vi "HDrive.Hashtag.vi"(2 "Percentage":dbl, 3 "Heading":dbl, 4 "X Input":dbl, 5 "Y Input":dbl) -> (0 "X Output":dbl, 1 "Y Output":dbl)   [LabVIEW 2014]
panel:
  out "Y-State":u16(ring) items=["Negative", "Positive"]
  out "X-State":u16(ring) items=["Negative", "Positive"]
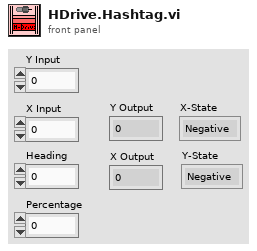
[diagram p1: front panel]
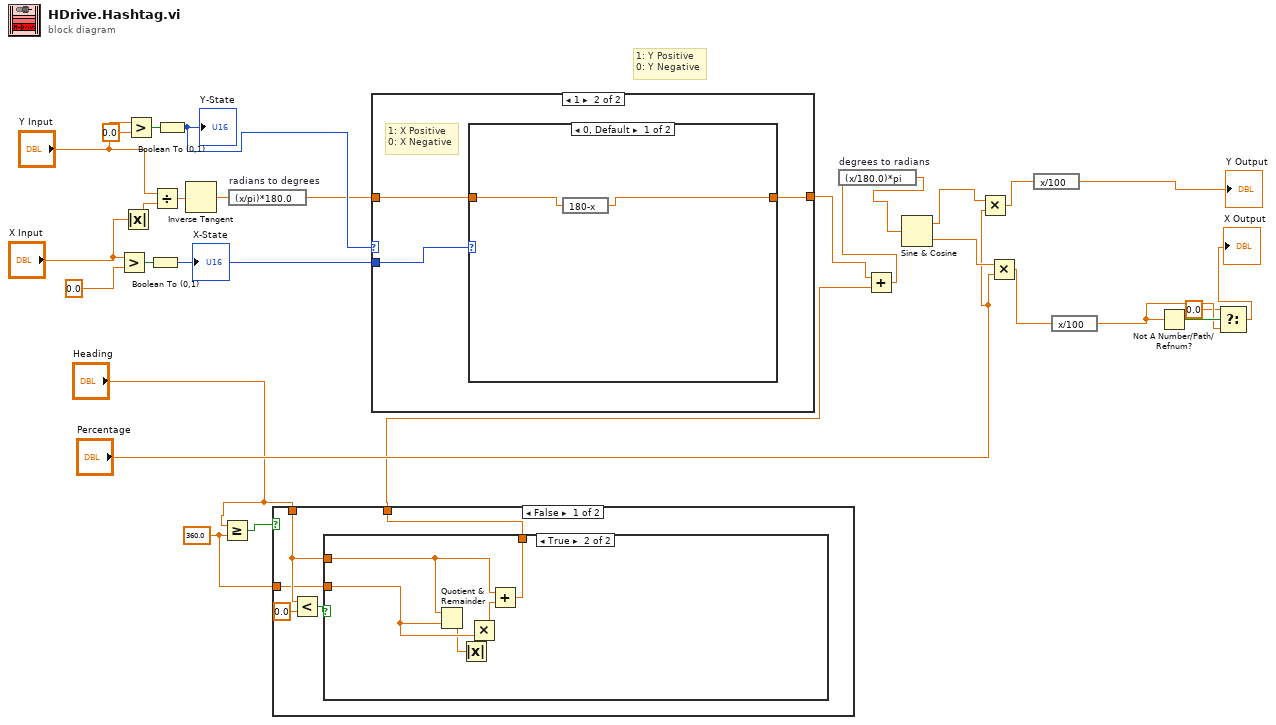
[diagram p0: block diagram]
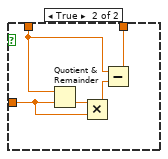
[diagram p3: hidden frame]
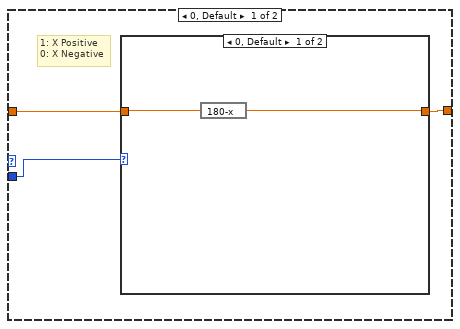
[diagram p4: hidden frame]
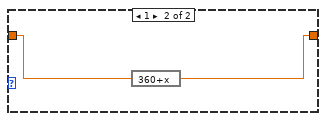
[diagram p5: hidden frame]
diagram:
  w8 = 360.0 ("y")
  # "1: Y Positive\n0: Y Negative"
  n1 = Greater?(x="X Input", y=0.0) -> (0:w27:bool)
  n2 = Absolute Value(x="X Input") -> (abs(x)=w28:dbl)
  n3 = Greater?(x="Y Input", y=0.0) -> (0:w24:bool)
  n4 = Boolean To (0,1)(Boolean=w27) -> (0, 1=w21:i16)
  "X-State" <- w21
  n5 = Divide(x="Y Input", y=w28) -> (x/y=w26:dbl)
  n6 = Boolean To (0,1)(Boolean=w24) -> (0, 1=w22:i16)
  "Y-State" <- w22
  n7 = Inverse Tangent(1:w26) -> (0:w25:dbl)
  n8 = Greater Or Equal?(x="Heading", y=w8) -> (x >= y?=w9:bool)
  n9 = expression code="(x/pi)*180.0" "radians to degrees"(w25) -> (w20:dbl)
  n10 = case shown="False" w9 {
    tunnel: "Heading" -> [w32 w44]
    tunnel: w8 -> [w31 w45]
    tunnel: [w30 w42] -> w6
    frame False {
      n11 = Less?(x=w32, y=0.0) -> (x < y?=w34:bool)
      n12 = case shown="True" w34 {
        tunnel: w32 -> [w35 w41]
        tunnel: w31 -> [_ w38]
        tunnel: [w35 w40] -> w30
        frame False {
        }
        frame True {
          n13 = Quotient & Remainder(x=w41, y=w38) -> (floor(x/y)=w37:dbl)  [unwired: 1 out]
          n14 = Absolute Value(x=w37) -> (abs(x)=w36:dbl)
          n15 = Multiply(x=w36, y=w38) -> (x*y=w39:dbl)
          n16 = Add(x=w41, y=w39) -> (x+y=w40:dbl)
        }
      }
    }
    frame True {
      n17 = Quotient & Remainder(x=w44, y=w45) -> (floor(x/y)=w46:dbl)  [unwired: 1 out]
      n18 = Multiply(x=w46, y=w45) -> (x*y=w43:dbl)
      n19 = Subtract(x=w44, y=w43) -> (x-y=w42:dbl)
    }
  }
  n20 = case shown="1" w22 {
    tunnel: w21 -> [w49 w56]
    tunnel: [w48 w55] -> w13
    tunnel: w20 -> [w47 w54]
    frame 0, Default {
      # "1: X Positive\n0: X Negative"
      n21 = case shown="0, Default" w49 {
        tunnel: [w50 w52] -> w48
        tunnel: w47 -> [w51 w53]
        frame 0, Default {
          n22 = expression code="180-x"(w51) -> (w50:dbl)
        }
        frame 1 {
          n23 = expression code="360+x"(w53) -> (w52:dbl)
        }
      }
    }
    frame 1 {
      # "1: X Positive\n0: X Negative"
      n24 = case shown="0, Default" w56 {
        tunnel: [w57 w59] -> w55
        tunnel: w54 -> [w58 w59]
        frame 0, Default {
          n25 = expression code="180-x"(w58) -> (w57:dbl)
        }
        frame 1 {
        }
      }
    }
  }
  n26 = Add(x=w13, y=w6) -> (x+y=w12:dbl)
  n27 = expression code="(x/180.0)*pi" "degrees to radians"(w12) -> (w17:dbl)
  n28 = Sine & Cosine(0:w17) -> (1:w16:dbl, 2:w15:dbl)
  n29 = Multiply(x=w16, y="Percentage") -> (x*y=w11:dbl)
  n30 = Multiply(x=w15, y="Percentage") -> (x*y=w10:dbl)
  n31 = expression code="x/100"(w11) -> (→"Y Output":dbl)
  n32 = expression code="x/100"(w10) -> (w3:dbl)
  n33 = Not A Number/Path/Refnum?(number/path/refnum=w3) -> (NaN/Path/Refnum?=w4:bool)
  n34 = Select(t=0.0, s=w4, f=w3) -> (s? t:f=→"X Output":dbl)
